vi "Get Data.vi"(8 "error in":errorcluster, 11 "Cfg Dev in":refnum<class "Vaisala.lvclass">) -> (0 "error out":errorcluster, 2 "Data":refnum<class "Data.lvclass">, 3 "Cfg Dev out":refnum<class "Vaisala.lvclass">)   [LabVIEW 2015, in "Vaisala.lvclass"]
uses:
  Vaisala.lvclass
  Reusable/Data/Data.lvclass
  Instruments/Nicholas/Session/FPGA Serial Session.lvclass
  Vaisala.lvclass/Vaisala.ctl
  Reusable/Data/Array Data/Single 1-D/Single_Array.lvclass
  Reusable/Data/Array Data/Single 1-D/Write Data.vi
  Reusable/Data/Write measTime.vi
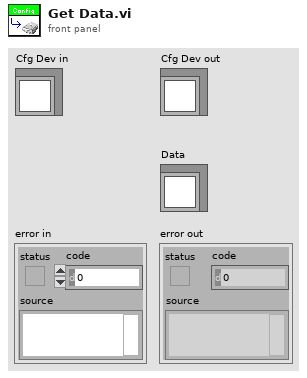
[diagram p1: front panel]
types:
  T1 = typedef "Session - Root.lvclass/Session Handle.ctl" = refnum<data-value>
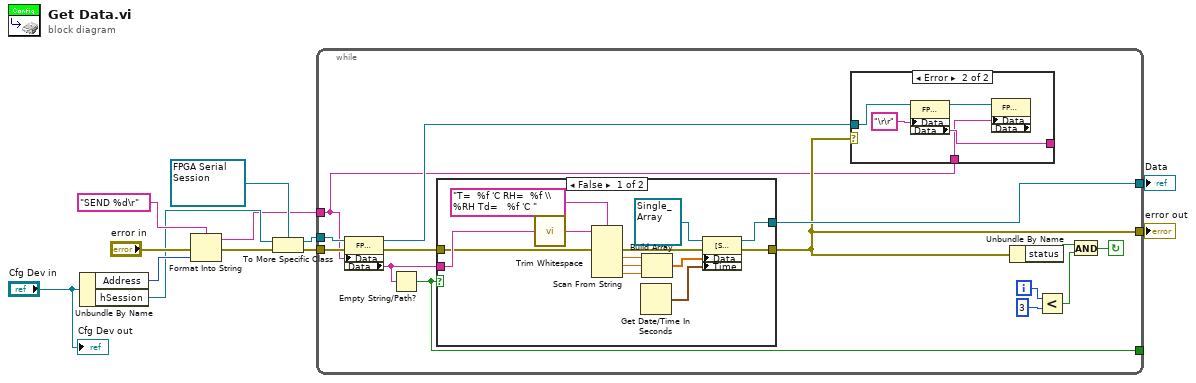
[diagram p0: block diagram]
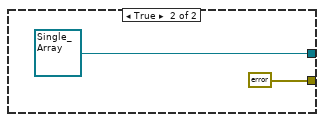
[diagram p3: hidden frame]
diagram:
  n1 = Unbundle By Name("Cfg Dev in") -> ("Address"=w11:u8, "hSession"=w4:T1)
  n2 = Format Into String(format string="SEND %d\r", error in="error in", w11) -> (resulting string=w1:string, error out=w6:errorcluster)  [unwired: 1 in]
  n3 = To More Specific Class(target class=refnum<data-value> refnum ("hSession"), reference=w4, error in=w6) -> (specific class reference=w8:refnum<data-value>, error out=w5:errorcluster)
  n4 = while {
    tunnel: w8 -> [w26]
    tunnel: w1 -> [w13]
    tunnel: [w16] -> _
    tunnel: [w18] -> w3
    tunnel: w5 -> [w25]
    tunnel: [w14] -> w2
    i -> [w24]
    stop <- w21 continue-if-true
    n5 = property class="FPGA Serial Session"(reference=w26, error in=w25, "Data"=w13) -> (reference out=w15:refnum<data-value>, error out=w20:errorcluster, "Data"=w19:string)
    n6 = Empty String/Path?(string/path=w19) -> (empty?=w16:bool)
    n7 = case shown="False" w16 {
      tunnel: w20 -> [w33 _]
      tunnel: [w43 refnum<class "Single_Array.lvclass"> refnum ("Base Data Class.lvlib:Single_Array.lvclass")] -> w18
      tunnel: [w41 errorcluster {"status"=TRUE, "code"=0, "source"=""} ("error out")] -> w14
      tunnel: w19 -> [w39 _]
      frame False {
        n8 = call <vilib>:"Trim Whitespace.vi"("string"=w39) -> ("trimmed string"=w38:string)  [unwired: 1 in]
        n9 = Scan From String(format string="T=  %f 'C RH=  %f \\%RH Td=   %f 'C ", input string=w38, error in=w33) -> (error out=w37:errorcluster, output 1=w36:dbl, output 2=w35:dbl, output 3=w34:dbl)  [unwired: 4 in, 2 out]
        n10 = Get Date/Time In Seconds() -> (seconds since 1Jan1904=w32:timestamp)
        n11 = Build Array(w36, w35, w34) -> (w42:dbl[])
        n12 = property class="[SGL]"(reference=refnum<class "Single_Array.lvclass"> refnum ("Base Data Class.lvlib:Single_Array.lvclass"), error in=w37, "Data"=w42, "Time"=w32) -> (reference out=w43:refnum<class "Single_Array.lvclass">, error out=w41:errorcluster)
      }
      frame True {
      }
    }
    n13 = case shown="Error" w14 {
      tunnel: w15 -> [_ w31]
      tunnel: [_ w29] -> _
      tunnel: w13 -> [_ w27]
      frame No Error {
      }
      frame Error {
        n14 = property class="FPGA Serial Session"(reference=w31, "Data"="\r\r") -> (reference out=w28:refnum<data-value>, "Data"=w29:string)  [unwired: 1 in, 1 out]
        n15 = property class="FPGA Serial Session" props=["Data", "Data"](reference=w28, "Data"=w27) -> ()  [unwired: 1 in, 3 out]
      }
    }
    n16 = Unbundle By Name(w14) -> ("status"=w17:bool)
    n17 = Less?(x=w24, y=3) -> (x < y?=w22:bool)
    n18 = And(x=w17, y=w22) -> (x .and. y?=w21:bool)
  }
  "error out" <- w2
  "Data" <- w3
  "Cfg Dev out" <- "Cfg Dev in"
